vi "LCR_TrimOC.vi"(8 "error in (no error)":errorcluster, 11 "WK6440B in":refnum<class "WK6440B.lvclass">) -> (0 "error out":errorcluster, 3 "WK6440B out":refnum<class "WK6440B.lvclass">)   [LabVIEW 2018, in "WK6440B.lvclass"]
uses:
  WK6440B.lvclass
  C:/Users/itk/Documents/itk-strip-sensor-qc/InstrControl/InstrControl.lvclass
  InstrControl.lvclass
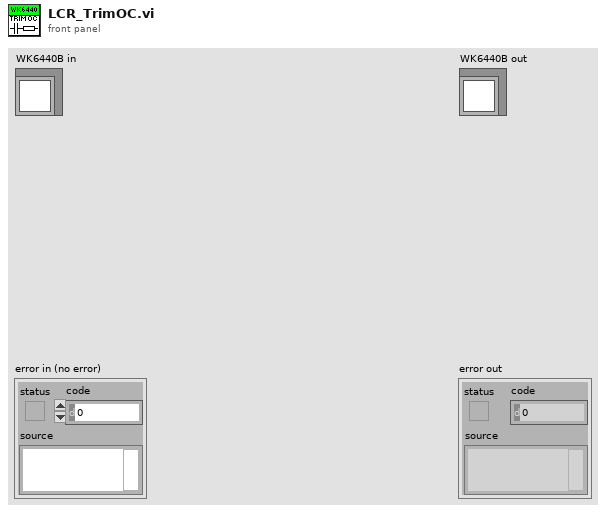
[diagram p1: front panel]
types:
  T1 = cluster{"error":bool, "code":i32, "source":string}
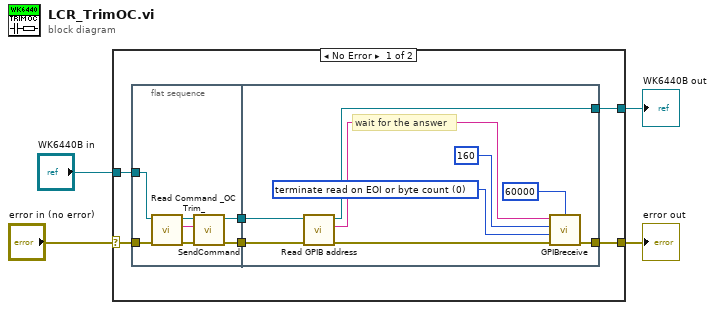
[diagram p0: block diagram]
diagram:
  n1 = case shown="No Error" "error in (no error)" {
    selector: "error in (no error)" -> [w9 w27]
    tunnel: "WK6440B in" -> [w10 w28]
    tunnel: [w6 w28] -> w2
    tunnel: [w5 w27] -> w1
    frame No Error {
      n2 = flat-sequence {
        tunnel: w10 -> [w17]
        tunnel: w9 -> [w16]
        tunnel: [w12] -> w8
        tunnel: [w11] -> w7
        tunnel: w8 -> [w26]
        tunnel: w7 -> [w20]
        tunnel: [w19] -> w6
        tunnel: [w18] -> w5
        frame #0 {
          n3 = call-dynamic "Read Command _OC Trim_.vi"("error in (no error)"=w16, "LCRControl in"=w17) -> ("error out"=w15:errorcluster, "Command \"OC Trim\""=w14:string, "LCRControl out"=w13:refnum<class "WK6440B.lvclass">)  [unwired: 7 in]
          n4 = call "SendCommand.vi"("error in (no error)"=w15, "Command string"=w14, "InstControl in"=w13) -> ("error out"=w11:errorcluster, "InstControl out"=w12:refnum<class "WK6440B.lvclass">)  [unwired: 7 in]
        }
        frame #1 {
          w23 = 0 items=["terminate read on EOI or byte count", "terminate read on EOI, byte count, or CR", "terminate read on EOI, byte count, or LF"] ("read mode")
          # "wait for the answer"
          n5 = call-dynamic "Read GPIB address.vi"("error in (no error)"=w20, "InstControl in"=w26) -> ("error out"=w21:errorcluster, "GPIB address"=w25:string, "InstControl out"=w19:refnum<class "WK6440B.lvclass">)  [unwired: 7 in]
          n6 = call "GPIBreceive.vi"("timeout ms"=u32 60000, "address string"=w25, "byte count"=160, "read mode"=w23, "error in"=w21) -> ("error out"=w18:T1)  [unwired: 2 in, 2 out]
        }
      }
    }
    frame Error {
    }
  }
  "error out" <- w1
  "WK6440B out" <- w2
